vi "LIEF Connector Main.vi"() -> ()   [LabVIEW 2016]
uses:
  Connector Editr Handler/Connector Editor Handler.lvclass
  C:/Program Files (x86)/National Instruments/LabVIEW 2016/vi.lib/LIEF/Image Editor Handler/Image Editor Handler.lvclass
  <vilib>/LIEF/Image Editor Handler/Image Editor Handler.lvclass/Image Editor Handler.ctl
  <vilib>/LIEF/Forms/Shape/Shape.lvclass/Shape.ctl
  <vilib>/LIEF/Forms/Layered Shape/Layered Shape.lvclass/Layered Shape.ctl
  <vilib>/LIEF/Image Editor Handler/Read Events.vi
  <vilib>/LIEF/Forms/Shape/Write Color.vi
  <vilib>/LIEF/Forms/Shape/Write Movable.vi
  <vilib>/LIEF/Forms/Layered Shape/Write Overlays.vi
  <vilib>/LIEF/Forms/Text/Text.lvclass
  C:/Program Files (x86)/National Instruments/LabVIEW 2016/vi.lib/LIEF/Forms/Shape/Shape.lvclass
  <vilib>/LIEF/Forms/Rectangle/Rectangle.lvclass
  C:/Program Files (x86)/National Instruments/LabVIEW 2016/vi.lib/LIEF/Forms/Layered Shape/Layered Shape.lvclass
  <vilib>/LIEF/Forms/Shape/Shape.lvclass
  <vilib>/LIEF/Image Editor Handler/Image Editor Handler.lvclass
  <vilib>/LIEF/Forms/Grid/Grid.lvclass
panel:
  in  "Connect":bool
  in  "2D Picture":picture
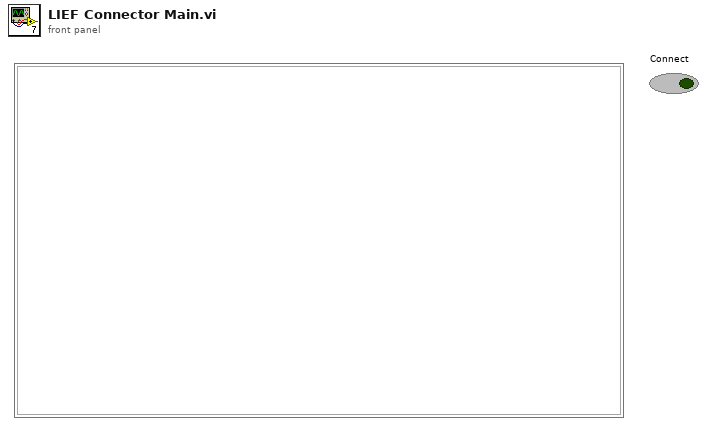
[diagram p1: front panel]
types:
  T1 = typedef "LVBoundsTypeDef.ctl" = cluster{"Width":u32, "Height":u32}
  T2 = enum16{"Left", "Top", "Right", "Bottom", "Centered"}
  T3 = typedef "LV Image Editor Framework.lvlib/Image Editor Handler.lvclass/Editor Events.ctl" = cluster{"Stop":refnum<user-event>, "Image Events":cluster{"AddShape":refnum<user-event>, "Paint":refnum<user-event>, "RemoveShape":refnum<user-event>, "RefreshShape ByRef":refnum<user-event>, "ShapePropertyChange":refnum<user-event>, "RemoveShape ByRef":refnum<user-event>}, "RequestShapes":refnum<user-event>, "Custom":refnum<user-event>}
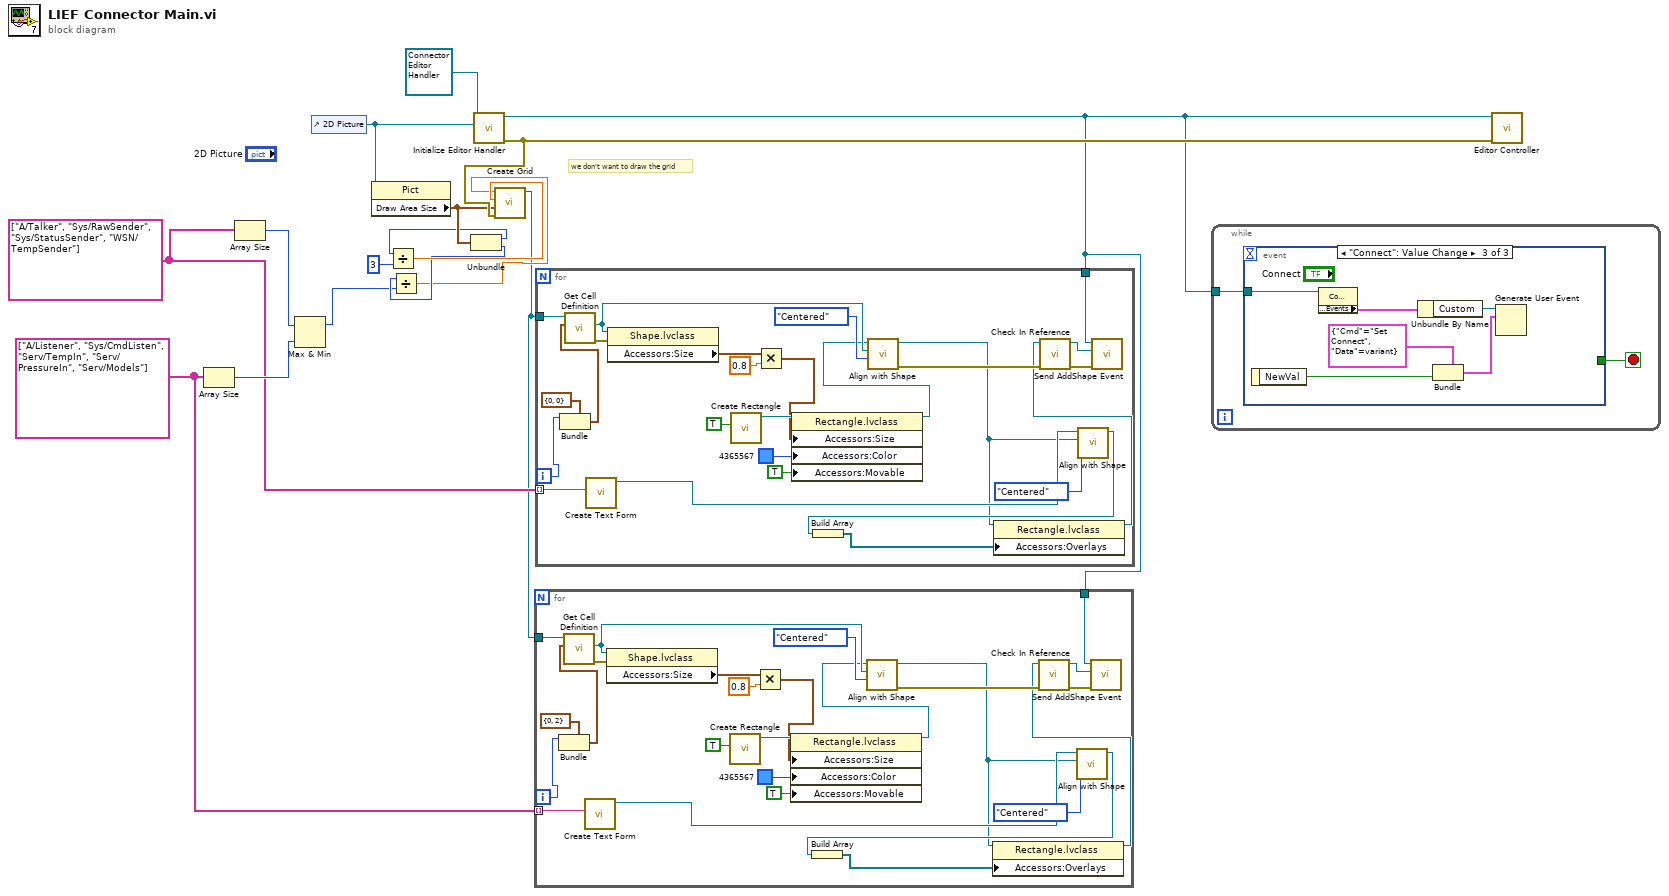
[diagram p0: block diagram]
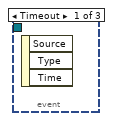
[diagram p2: hidden frame]
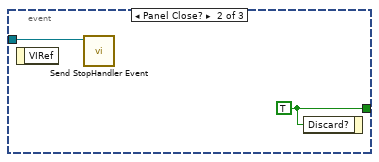
[diagram p3: hidden frame]
diagram:
  w1 = string[] ["A/Listener", "Sys/CmdListen", "Serv/TempIn", "Serv/PressureIn", "Serv/Models"]
  w4 = string[] ["A/Talker", "Sys/RawSender", "Sys/StatusSender", "WSN/TempSender"]
  # "we don't want to draw the grid"
  n1 = Array Size(array=w1) -> (size(s)=w12:i32)
  n2 = Array Size(array=w4) -> (size(s)=w13:i32)
  n3 = Max & Min(x=w13, y=w12) -> (max(x,y)=w6:i32)  [unwired: 1 out]
  n4 = control-ref of="2D Picture"() -> (w16:refnum<vi>)
  n5 = property class="Pict"(reference=w16) -> ("Draw Area Size"=w10:T1)  [unwired: 1 in, 2 out]
  n6 = Unbundle(w10) -> ("Width"=w9:u32, "Height"=w7:u32)
  n7 = Divide(x=w9, y=3) -> (x/y=w8:dbl)
  n8 = Divide(x=w7, y=w6) -> (x/y=w5:dbl)
  n9 = call <vilib>:"Initialize Editor Handler.vi"("PictureRef"=w16, "Editor Handler in"=refnum<class "Connector Editor Handler.lvclass"> refnum ("Connector Editor Handler.lvclass")) -> ("error out"=w15:errorcluster, "Editor Handler out"=w2:refnum<class "Connector Editor Handler.lvclass">)  [unwired: 8 in]
  n10 = call <vilib>:"Create Grid.vi"("error in (no error)"=w15, "Draw Area"=w10, "Horizontal Step"=w8, "Vertical Step"=w5) -> ("Grid Reference"=w3:refnum<data-value>)  [unwired: 6 in, 1 out]
  n11 = for {
    tunnel: w3 -> [w42]
    tunnel: w2 -> [w35]
    tunnel: w1 -> [w24] mode=indexing
    i -> [w26]
    n12 = Bundle(cluster=cluster{"Row":u32, "Column":i32} {"Row"=0, "Column"=2} ("Indexes"), "Row"=w26) -> (w25:cluster{"Row":u32, "Column":i32})  [unwired: 1 in]
    n13 = call <vilib>:"Get Cell Definition.vi"("Indexes"=w25, "Shape Reference"=w42) -> ("error out"=w40:errorcluster, "Cell"=w39:refnum<class "Shape.lvclass">)  [unwired: 7 in, 1 out]
    n14 = call <vilib>:"Create Text Form.vi"("Text"=w24) -> ("New Text"=w23:refnum<class "Text.lvclass">)  [unwired: 9 in, 1 out]
    n15 = property class="Shape.lvclass"(reference=w39, error in=w40) -> ("Accessors:Size"=w38:cluster{"Width":i32, "Height":i32})  [unwired: 2 out]
    n16 = call <vilib>:"Create Rectangle.vi"("Filled"=TRUE) -> ("Rectangle out"=w32:refnum<class "Rectangle.lvclass">)  [unwired: 9 in, 1 out]
    n17 = Multiply(x=w38, y=0.8) -> (x*y=w31:cluster{"Width":dbl, "Height":dbl})
    n18 = property class="Rectangle.lvclass"(reference=w32, "Accessors:Size"=w31, "Accessors:Color"=u32 4365567 ("Color"), "Accessors:Movable"=TRUE ("Movable")) -> (reference out=w19:refnum<class "Rectangle.lvclass">)  [unwired: 1 in, 1 out]
    n19 = call <vilib>:"Align with Shape.vi"("Alignment"=T2."Centered", "Reference Shape"=w39, "Shape in"=w19) -> ("error out"=w34:errorcluster, "Shape out"=w17:refnum<class "Rectangle.lvclass">)  [unwired: 7 in]
    n20 = call <vilib>:"Align with Shape.vi"("Alignment"=T2."Centered", "Reference Shape"=w17, "Shape in"=w23) -> ("Shape out"=w21:refnum<class "Text.lvclass">)  [unwired: 7 in, 1 out]
    n21 = Build Array(w21) -> (w20:refnum<class "Text.lvclass">[])
    n22 = property class="Rectangle.lvclass"(reference=w17, "Accessors:Overlays"=w20) -> (reference out=w18:refnum<class "Rectangle.lvclass">)  [unwired: 1 in, 1 out]
    n23 = call <vilib>:"Check In Reference.vi"("error in (no error)"=w34, "Shape in"=w18) -> ("error out"=w33:errorcluster, "Shape Reference"=w36:refnum<data-value>)  [unwired: 8 in]
    n24 = call <vilib>:"Send AddShape Event.vi"("error in (no error)"=w33, "New Shape Reference"=w36, "Editor Handler in"=w35) -> ()  [unwired: 7 in, 2 out]
  }
  n25 = for {
    tunnel: w3 -> [w68]
    tunnel: w2 -> [w61]
    tunnel: w4 -> [w50] mode=indexing
    i -> [w52]
    n26 = Bundle(cluster=cluster{"Row":u32, "Column":u32} {"Row"=0, "Column"=0} ("Indexes"), "Row"=w52) -> (w51:cluster{"Row":u32, "Column":u32})  [unwired: 1 in]
    n27 = call <vilib>:"Get Cell Definition.vi"("Indexes"=w51, "Shape Reference"=w68) -> ("error out"=w66:errorcluster, "Cell"=w65:refnum<class "Shape.lvclass">)  [unwired: 7 in, 1 out]
    n28 = call <vilib>:"Create Text Form.vi"("Text"=w50) -> ("New Text"=w49:refnum<class "Text.lvclass">)  [unwired: 9 in, 1 out]
    n29 = property class="Shape.lvclass"(reference=w65, error in=w66) -> ("Accessors:Size"=w64:cluster{"Width":i32, "Height":i32})  [unwired: 2 out]
    n30 = call <vilib>:"Create Rectangle.vi"("Filled"=TRUE) -> ("Rectangle out"=w58:refnum<class "Rectangle.lvclass">)  [unwired: 9 in, 1 out]
    n31 = Multiply(x=w64, y=0.8) -> (x*y=w57:cluster{"Width":dbl, "Height":dbl})
    n32 = property class="Rectangle.lvclass"(reference=w58, "Accessors:Size"=w57, "Accessors:Color"=u32 4365567 ("Color"), "Accessors:Movable"=TRUE ("Movable")) -> (reference out=w45:refnum<class "Rectangle.lvclass">)  [unwired: 1 in, 1 out]
    n33 = call <vilib>:"Align with Shape.vi"("Alignment"=T2."Centered", "Reference Shape"=w65, "Shape in"=w45) -> ("error out"=w60:errorcluster, "Shape out"=w43:refnum<class "Rectangle.lvclass">)  [unwired: 7 in]
    n34 = call <vilib>:"Align with Shape.vi"("Alignment"=T2."Centered", "Reference Shape"=w43, "Shape in"=w49) -> ("Shape out"=w47:refnum<class "Text.lvclass">)  [unwired: 7 in, 1 out]
    n35 = Build Array(w47) -> (w46:refnum<class "Text.lvclass">[])
    n36 = property class="Rectangle.lvclass"(reference=w43, "Accessors:Overlays"=w46) -> (reference out=w44:refnum<class "Rectangle.lvclass">)  [unwired: 1 in, 1 out]
    n37 = call <vilib>:"Check In Reference.vi"("error in (no error)"=w60, "Shape in"=w44) -> ("error out"=w59:errorcluster, "Shape Reference"=w62:refnum<data-value>)  [unwired: 8 in]
    n38 = call <vilib>:"Send AddShape Event.vi"("error in (no error)"=w59, "New Shape Reference"=w62, "Editor Handler in"=w61) -> ()  [unwired: 7 in, 2 out]
  }
  n39 = while {
    tunnel: w2 -> [w69]
    stop <- w70 stop-if-true
    n40 = event shown="[2] \"Connect\": Value Change" {
      selector: _ -> [_ _ _]
      dyn-events: _ -> [_ _ _]
      timeout: _ -> [_ _ _]
      tunnel: [_ w72 _] -> w70
      tunnel: w69 -> [_ w71 w74]
      event Timeout {
        n41 = event-data() -> ()  [unwired: 1 in, 3 out]
      }
      event Panel Close? {
        w72 = TRUE ("Discard?")
        n42 = event-data() -> ()  [unwired: 1 in, 1 out]
        n43 = call <vilib>:"Send StopHandler Event.vi"("Editor Handler in"=w71) -> ()  [unwired: 9 in, 2 out]
        n44 = event-data("Discard?"=w72) -> ()  [unwired: 1 in, 1 out]
      }
      event "Connect": Value Change {
        n45 = event-data() -> ("NewVal"=w76:bool)  [unwired: 1 in]
        n46 = property class="Connector Editor Handler.lvclas"(reference=w74) -> ("Accessors:Events"=w75:T3)  [unwired: 1 in, 2 out]
        n47 = Unbundle By Name(w75) -> ("Custom"=w73:refnum<user-event>)
        n48 = Bundle(cluster=cluster{"Cmd":string, "Data":variant} {"Cmd"="Set Connect", "Data"=variant} ("event data"), "Data"=w76) -> (w77:cluster{"Cmd":string, "Data":variant})  [unwired: 1 in]
        n49 = Generate User Event(user event=w73, event data cluster=w77) -> ()  [unwired: 2 in, 2 out]
      }
    }
  }
  n50 = call <vilib>:"Editor Controller.vi"("error in (no error)"=w15, "Editor Handler in"=w2) -> ()  [unwired: 8 in, 2 out]
